vi "Rising Edge Trigger.vi"(1 "Signal":bool) -> (0 "Trigger?":bool)   [LabVIEW 2018]
doc: "A rising edge of the <b>Input Signal</b> is triggered with the condition that the previous value is FALSE and the current value is TRUE."
panel:
  # "A rising edge of the Input Signal is triggered with the condition that the previous value is FALSE and the current value is TRUE."
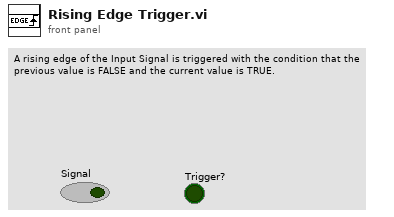
[diagram p1: front panel]
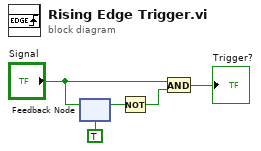
[diagram p0: block diagram]
diagram:
  n1 = feedback #1(TRUE ("Signal")) -> (w4:bool)
  n2 = feedback-in #1("Signal") -> ()
  n3 = Not(x=w4) -> (.not. x?=w3:bool)
  n4 = And(x="Signal", y=w3) -> (x .and. y?=→"Trigger?":bool)
